vi "RF mapping_flash.vi"() -> ()   [LabVIEW 2013]
uses:
  <vilib>/Platform/TimedLoop/XDataNode/timing_clust.ctl
  <vilib>/Platform/TimedLoop/XDataNode/nitl_modes.ctl
  <vilib>/Platform/TimedLoop/XDataNode/wakeup.ctl
  Eye tracking dependencies/Global 1.vi
  <vilib>/platform/TimedLoop/XDataNode/XDataNode.xnode
  <vilib>/Platform/TimedLoop/XDataNode/XDNodeRunTimeDep.lvlib
panel:
  out "VS missed!":bool
  out "Originating IP":string="192.168.137.2"
  out "Incoming data":string="TrlDone 5.000 "
  out "Current trial":u16=9091
  in  "Trials":u16=2
  in  "Stop flashing":bool=TRUE
  out "VS busy":bool
  in  "Update cycle (ms)":dbl=50.0
  in  "VS subtype":string="20x14"
  in  "VS type":string="RF_mapping"
  in  "Remote port":u16=9091
  in  "Local port":u16=9090
  in  "Remote IP - Broadcast":string="192.168.137.255"
  in  "Remote IP - VS":string="192.168.137.3"
  in  "Local IP - this computer":string="192.168.137.10"
  in  "Mean luminance":sgl=40.0 format="%#_13g"
  in  "Inter trial interval (s)":sgl=1.0 format="%#_13g"
  in  "After VS (s)":sgl format="%#_13g"
  in  "Before VS (s) - not used":sgl format="%#_13g"
  in  "Inter flash interval (s)":sgl=0.3 format="%#_13g"
  in  "ON duration (s)":sgl=0.032 format="%#_13g"
  in  "OFF duration (s)":sgl=0.032 format="%#_13g"
  in  "Stop the VI":bool=TRUE
  in  "Start flashing":bool=TRUE
  # "Receptive field mapping with flashing squares"
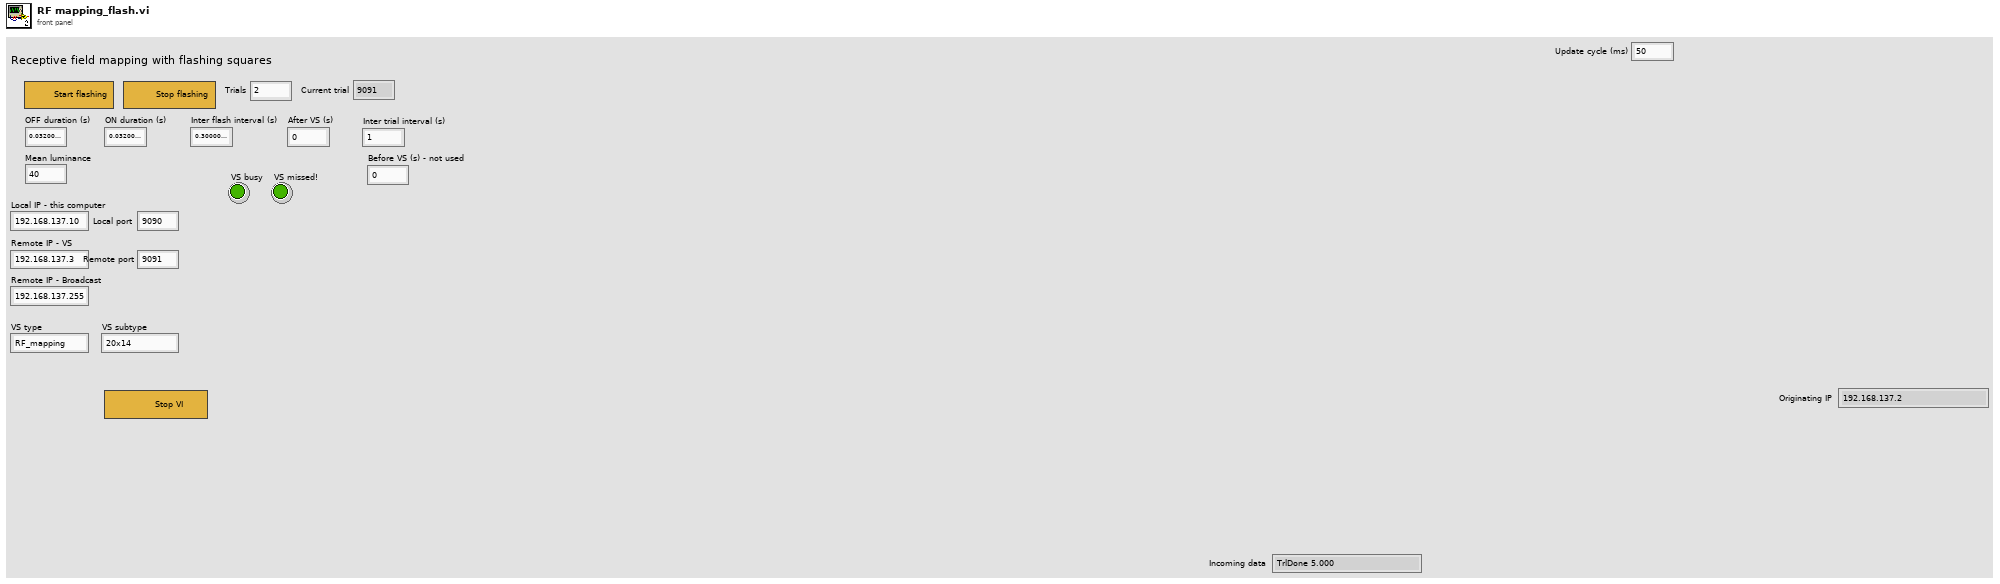
[diagram p1: front panel]
types:
  T1 = typedef "XDNodeRunTimeDep.lvlib/timing_clust.ctl" = cluster{"Expected End [f-1]":u64, "Actual End [f-1]":u64, "Finished Late? [f-1]":bool, "Expected End [i-1]":u64, "Actual End [i-1]":u64, "Finished Late? [i-1]":bool, "Expected Start [i]":u64, "Actual Start [i]":u64, "Expected Start [f]":u64, "Actual Start [f]":u64, "Source Name":string, "Structure Name":string, "Period":i64, "Deadline":i64, "Offset":i64, "Start":i64, "Priority":i32, "Timeout":i32, "Mode":T2, "Wakeup Reason":T3, "Error":errorcluster, "Source Type":string, "Secondary Source Type":string, "Global End Time":u64, "Global Start Time":u64, "Frame Duration":u64, "Iteration Duration":u64, "Assigned CPU":i32, "I/O Scan Engine Mode":u32}
  T2 = typedef "XDNodeRunTimeDep.lvlib/nitl_modes.ctl" = enum32{"No Change", "Process missed periods, maintain original phase", "Discard missed periods, maintain original phase", "Process missed periods, ignore original phase", "Discard missed periods, ignore original phase"}
  T3 = typedef "XDNodeRunTimeDep.lvlib/wakeup.ctl" = enum32{"Normal", "Aborted", "Asynchronous wakeup", "Timing source error", "Timed loop error", "Timeout"}
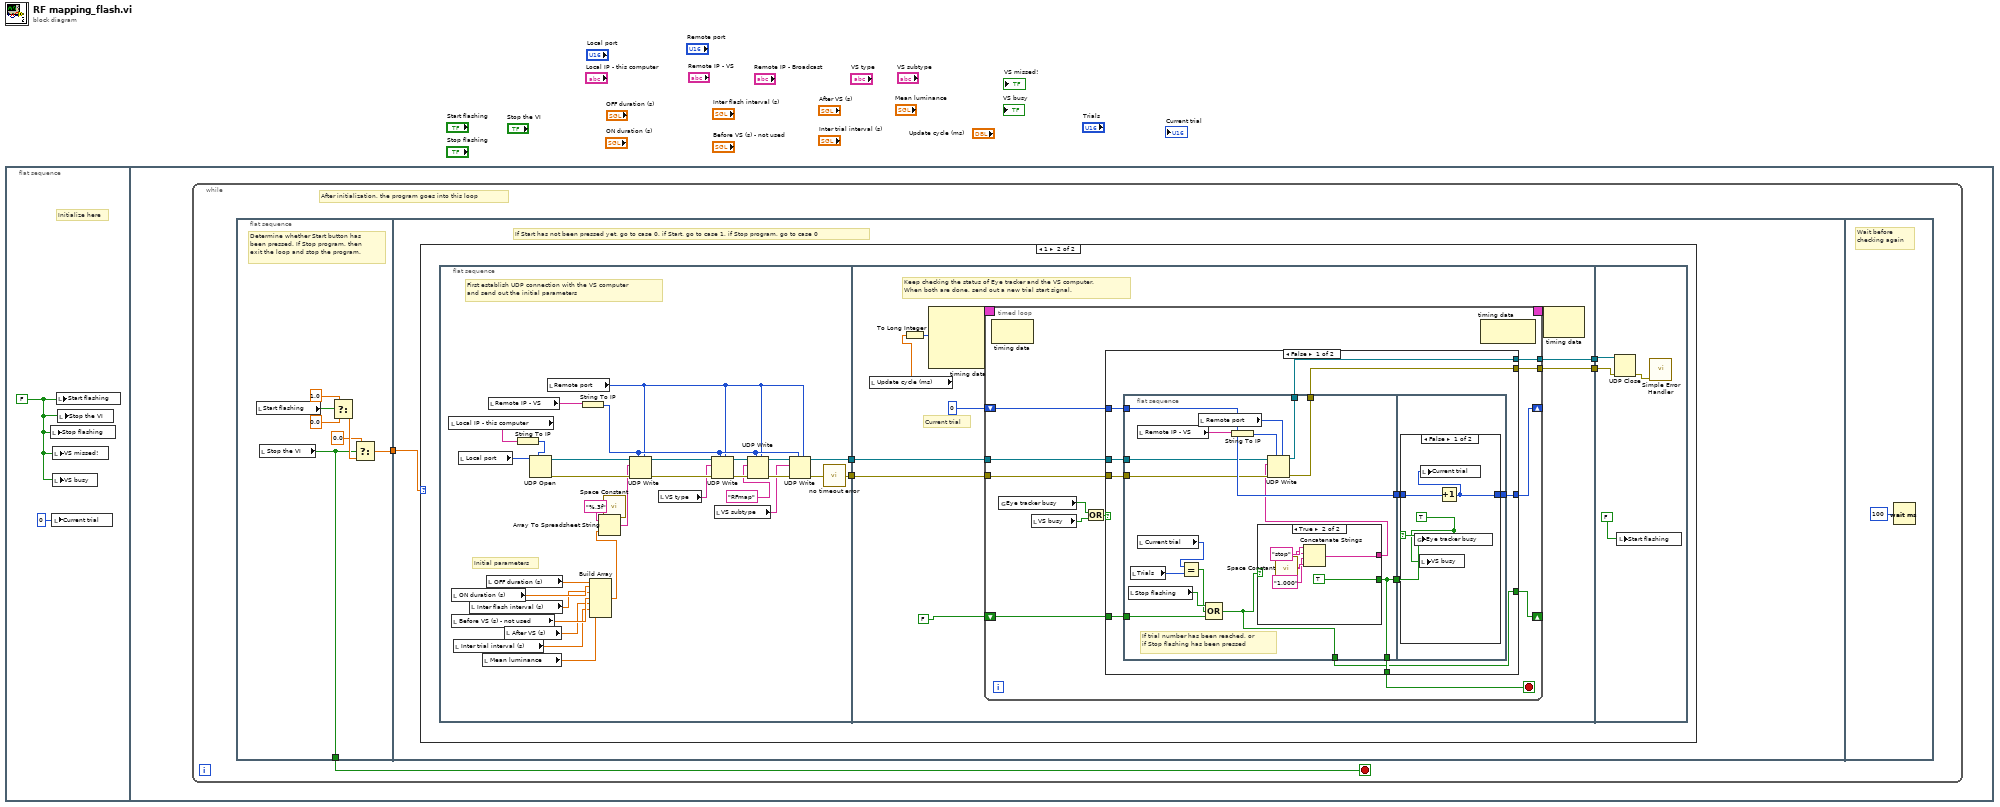
[diagram p0: block diagram]
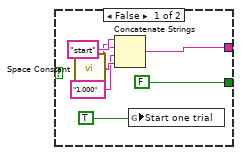
[diagram p3: hidden frame]
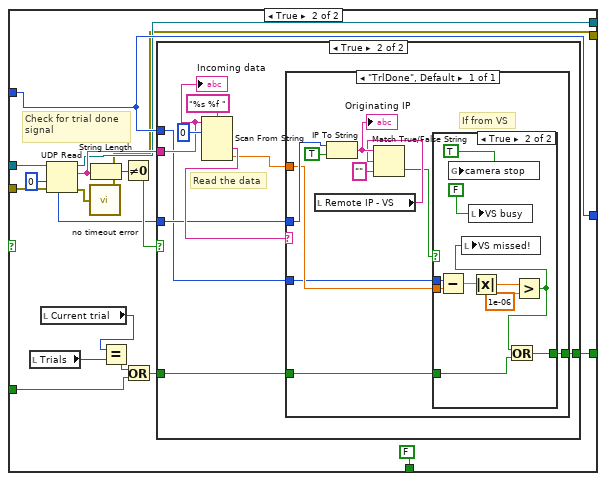
[diagram p5: hidden frame]
diagram:
  n1 = flat-sequence {
    frame #0 {
      w2 = FALSE
      # "Initialize here"
      n2 = local write "Stop flashing"(w2) -> ()
      n3 = local write "Current trial"(u16 0 ("Current trial")) -> ()
      n4 = local write "VS missed!"(w2) -> ()
      n5 = local write "VS busy"(w2) -> ()
      n6 = local write "Start flashing"(w2) -> ()
      n7 = local write "Stop the VI"(w2) -> ()
    }
    frame #1 {
      n8 = while {
        stop <- w3 stop-if-true
        # "After initialization, the program goes into this loop"
        n9 = flat-sequence {
          tunnel: [w6] -> w4
          tunnel: [w5] -> w3
          tunnel: w4 -> [w12]
          frame #0 {
            # "Determine whether Start button has \nbeen pressed. If Stop program, then \nexit the loop and stop the program."
            n10 = local read "Start flashing"() -> (w11:bool)
            n11 = local read "Stop the VI"() -> (w5:bool)
            n12 = Select(t=1.0, s=w11, f=0.0) -> (s? t:f=w8:dbl)
            n13 = Select(t=0.0, s=w5, f=w8) -> (s? t:f=w6:dbl)
          }
          frame #1 {
            # "If Start has not been pressed yet, go to case 0, if Start, go to case 1, if Stop program, go to case 0"
            n14 = case shown="1" w12 {
              frame 0, Default {
              }
              frame 1 {
                n15 = flat-sequence {
                  tunnel: [w18] -> w16
                  tunnel: [w17] -> w15
                  tunnel: w16 -> [w53]
                  tunnel: w15 -> [w52]
                  tunnel: [w49] -> w14
                  tunnel: [w48] -> w13
                  tunnel: w14 -> [w173]
                  tunnel: w13 -> [w172]
                  frame #0 {
                    # "Initial parameters"
                    # "First establish UDP connection with the VS computer\nand send out the initial parameters"
                    n16 = local read "Local IP - this computer"() -> (w47:string)
                    n17 = local read "ON duration (s)"() -> (w38:sgl)
                    n18 = local read "Before VS (s) - not used"() -> (w36:sgl)
                    n19 = local read "Inter trial interval (s)"() -> (w34:sgl)
                    n20 = local read "Local port"() -> (w46:u16)
                    n21 = local read "Inter flash interval (s)"() -> (w37:sgl)
                    n22 = local read "Mean luminance"() -> (w33:sgl)
                    n23 = local read "OFF duration (s)"() -> (w39:sgl)
                    n24 = local read "Remote IP - VS"() -> (w44:string)
                    n25 = local read "After VS (s)"() -> (w35:sgl)
                    n26 = String To IP(1:w47) -> (0:w45:u32)
                    n27 = UDP Open(7:w45, 11:w46) -> (port=w43:refnum<k16>, 0:w42:errorcluster)  [unwired: 3 in, 1 out]
                    n28 = local read "Remote port"() -> (w20:u16)
                    n29 = String To IP(1:w44) -> (0:w21:u32)
                    n30 = Build Array(w39, w38, w37, w36, w35, w34, w33) -> (w32:sgl[])
                    n31 = call <vilib>:"Space Constant.vi"() -> ("String"=w41:string)
                    n32 = Array To Spreadsheet String(delimiter (Tab)=w41, array=w32, 3:"%.3f" ("format string")) -> (spreadsheet string=w31:string)
                    n33 = UDP Write(address=w21, port or service name=w20, connection ID=w43, data in=w31, 8:w42) -> (error out=w30:errorcluster, 3:w29:refnum<k16>)  [unwired: 1 in]
                    n34 = local read "VS type"() -> (w28:string)
                    n35 = UDP Write(address=w21, port or service name=w20, connection ID=w29, data in=w28, 8:w30) -> (error out=w27:errorcluster, 3:w26:refnum<k16>)  [unwired: 1 in]
                    n36 = local read "VS subtype"() -> (w22:string)
                    n37 = UDP Write(address=w21, port or service name=w20, connection ID=w26, data in="RFmap", 8:w27) -> (error out=w24:errorcluster, 3:w23:refnum<k16>)  [unwired: 1 in]
                    n38 = UDP Write(address=w21, port or service name=w20, connection ID=w23, data in=w22, 8:w24) -> (error out=w19:errorcluster, 3:w18:refnum<k16>)  [unwired: 1 in]
                    n39 = call "no timeout error.vi"("error in (no error)"=w19) -> ("error out"=w17:errorcluster)
                  }
                  frame #1 {
                    # "Current trial"
                    # "Keep checking the status of Eye tracker and the VS computer.\nWhen both are done, send out a new trial start signal."
                    n40 = local read "Update cycle (ms)"() -> (w55:dbl)
                    n41 = To Long Integer(number=w55) -> (32bit integer=w54:i32)
                    n42 = node-c288(w54) -> (w57:T1)  [unwired: 3 in]
                    n43 = timed-loop {
                      timing: w57 -> [_]
                      timing-out: [_] -> w56
                      tunnel: w53 -> [w66]
                      tunnel: w52 -> [w65]
                      shift-right: [w62] -> _
                      shift-left: 0 -> [w63]
                      shift-right: [w60] -> _
                      shift-left: FALSE -> [w61]
                      tunnel: [w59] -> w49
                      tunnel: [w58] -> w48
                      stop <- w64 stop-if-true
                      n44 = node-c288() -> ()  [unwired: 1 in, 1 out]
                      n45 = global read "Global 1.vi" "Eye tracker busy"() -> (w68:bool)
                      n46 = local read "VS busy"() -> (w69:bool)
                      n47 = Or(x=w68, y=w69) -> (x .or. y?=w67:bool)
                      n48 = case shown="False" w67 {
                        tunnel: w66 -> [w77 w130]
                        tunnel: w65 -> [w76 w131]
                        tunnel: [w80 FALSE] -> w64
                        tunnel: w63 -> [w78 w123]
                        tunnel: [w74 w123] -> w62
                        tunnel: w61 -> [w73 w119]
                        tunnel: [w72 w117] -> w60
                        tunnel: [w71 w116] -> w59
                        tunnel: [w70 w115] -> w58
                        frame False {
                          n49 = flat-sequence {
                            tunnel: [w86] -> w80
                            tunnel: [w94] -> w79
                            tunnel: w78 -> [w94]
                            tunnel: w77 -> [w92]
                            tunnel: w76 -> [w91]
                            tunnel: [w86] -> w75
                            tunnel: w73 -> [w84]
                            tunnel: [w83] -> w72
                            tunnel: [w82] -> w71
                            tunnel: [w81] -> w70
                            tunnel: w79 -> [w109]
                            tunnel: w75 -> [w110]
                            tunnel: [w108] -> w74
                            frame #0 {
                              # "If trial number has been reached, or \nif Stop flashing has been pressed"
                              n50 = local read "Stop flashing"() -> (w96:bool)
                              n51 = local read "Trials"() -> (w95:u16)
                              n52 = local read "Remote IP - VS"() -> (w90:string)
                              n53 = local read "Current trial"() -> (w85:u16)
                              n54 = Equal?(x=w85, y=w95) -> (x = y?=w93:bool)
                              n55 = local read "Remote port"() -> (w88:u16)
                              n56 = Compound Arithmetic op=OR(w96, w93, w84) -> (w83:bool)
                              n57 = String To IP(1:w90) -> (0:w89:u32)
                              n58 = case shown="True" w83 {
                                tunnel: [w99 w104] -> w87
                                tunnel: [FALSE TRUE] -> w86
                                frame False {
                                n59 = call <vilib>:"Space Constant.vi"() -> ("String"=w101:string)
                                n60 = Concatenate Strings("start", w101, "1.000", w101) -> (w99:string)
                                n61 = global write "Global 1.vi" "Start one trial"(TRUE) -> ()
                                }
                                frame True {
                                n62 = call <vilib>:"Space Constant.vi"() -> ("String"=w106:string)
                                n63 = Concatenate Strings("stop", w106, "1.000", w106) -> (w104:string)
                                }
                              }
                              n64 = UDP Write(address=w89, port or service name=w88, connection ID=w92, data in=w87, 8:w91) -> (error out=w81:errorcluster, 3:w82:refnum<k16>)  [unwired: 1 in]
                            }
                            frame #1 {
                              n65 = case shown="False" w110 {
                                tunnel: w109 -> [w113 w114]
                                tunnel: [w111 w114] -> w108
                                frame False {
                                w112 = TRUE
                                n66 = global write "Global 1.vi" "Eye tracker busy"(w112) -> ()
                                n67 = local write "VS busy"(w112) -> ()
                                n68 = Increment(x=w113) -> (x+1=w111:i32)
                                n69 = local write "Current trial"(w111) -> ()
                                }
                                frame True {
                                }
                              }
                            }
                          }
                        }
                        frame True {
                          # "Check for trial done\nsignal"
                          n70 = local read "Trials"() -> (w122:u16)
                          n71 = local read "Current trial"() -> (w121:u16)
                          n72 = UDP Read(connection ID=w130, timeout ms (25000)=0, 8:w131) -> (data out=w125:string, error out=w127:errorcluster, 3:w116:refnum<k16>, 6:w124:u32)  [unwired: 1 in, 1 out]
                          n73 = call "no timeout error.vi"("error in (no error)"=w127) -> ("error out"=w115:errorcluster)
                          n74 = String Length(string=w125) -> (length=w129:i32)
                          n75 = Equal?(x=w121, y=w122) -> (x = y?=w120:bool)
                          n76 = Not Equal To 0?(x=w129) -> (x != 0?=w126:bool)
                          n77 = Or(x=w120, y=w119) -> (x .or. y?=w118:bool)
                          n78 = case shown="True" w126 {
                            tunnel: w125 -> [_ w140]
                            tunnel: w124 -> [_ w138]
                            tunnel: w123 -> [_ w136]
                            tunnel: w118 -> [w133 w135]
                            tunnel: [w133 w134] -> w117
                            frame False {
                            }
                            frame True {
                              # "Read the data"
                              n79 = Scan From String(format string="%s %f ", input string=w140, initial scan location=u32 0) -> (output 1=w139:string, output 2=w137:dbl)  [unwired: 3 in, 3 out]
                              n80 = case shown="\"TrlDone\", Default" w139 {
                                tunnel: w138 -> [w149]
                                tunnel: w137 -> [w146]
                                tunnel: w136 -> [w145]
                                tunnel: w135 -> [w144]
                                tunnel: [w143] -> w134
                                frame "TrlDone", Default {
                                # "If from VS"
                                n81 = local read "Remote IP - VS"() -> (w148:string)
                                n82 = IP To String(1:TRUE ("dot notation? (F)"), 2:w149) -> (0:w150:string)
                                "Originating IP" <- w150
                                n83 = Match True/False String(2:"" ("false string"), 3:w148, 4:w150) -> (0:w147:bool)  [unwired: 1 out]
                                n84 = case shown="True" w147 {
                                tunnel: w146 -> [_ w160]
                                tunnel: w145 -> [_ w159]
                                tunnel: w144 -> [w153 w156]
                                tunnel: [w153 w155] -> w143
                                frame False {
                                }
                                frame True {
                                n85 = Subtract(x=w159, y=w160) -> (x-y=w161:dbl)
                                n86 = global write "Global 1.vi" "camera stop"(TRUE ("dot notation? (F)")) -> ()
                                n87 = local write "VS busy"(FALSE) -> ()
                                n88 = Absolute Value(x=w161) -> (abs(x)=w162:dbl)
                                n89 = Greater?(x=w162, y=1e-06) -> (0:w157:bool)
                                n90 = local write "VS missed!"(w157) -> ()
                                n91 = Or(x=w157, y=w156) -> (x .or. y?=w155:bool)
                                }
                                }
                                }
                              }
                              "Incoming data" <- w140
                            }
                          }
                        }
                      }
                      n92 = node-c288() -> ()  [unwired: 1 in, 1 out]
                    }
                    n93 = node-c288(w56) -> ()  [unwired: 1 out]
                  }
                  frame #2 {
                    n94 = UDP Close(connection ID=w173, 8:w172) -> (error out=w171:errorcluster)  [unwired: 1 out]
                    n95 = local write "Start flashing"(FALSE) -> ()
                    n96 = call <vilib>:"Simple Error Handler.vi"("error in (no error)"=w171) -> ()  [unwired: 4 in, 5 out]
                  }
                }
              }
            }
          }
          frame #2 {
            # "Wait before \nchecking again"
            n97 = Wait (ms)(milliseconds to wait=u32 100) -> ()  [unwired: 1 out]
          }
        }
      }
    }
  }
